vi "Configure Trigger.vi"(8 "error in (no error)":errorcluster, 11 "Thermometer DAQmx Base CFG in":refnum<class "Thermometer DAQmx Base CFG.lvclass">) -> (0 "error out":errorcluster, 3 "Thermometer DAQmx Base CFG out":refnum<class "Thermometer DAQmx Base CFG.lvclass">)   [LabVIEW 2023, in "Thermometer DAQmx Base CFG.lvlib" / "Thermometer DAQmx Base CFG.lvclass"]
uses:
  Thermometer DAQmx Base CFG.lvclass
  Thermometer DAQmx Base CFG.lvclass/Thermometer DAQmx Base CFG.ctl
  1ef251c9-8369-4278-8302-97e96edc9e10.vi
  <vilib>/ErrorRing/Error Ring.xnode
  <vilib>/JDP Science/JSONtext/JSONtext.lvlib
  <vilib>/Utility/error.llb/Error Cluster From Error Code.vi
  Configuration JSON Base/CFG JSON Base.lvclass
  D:/git/HAL/HAL GOOP4/Configuration JSON Base/CFG JSON Base.lvclass
  D:/git/HAL/HAL GOOP4/Interfaces/IConfigure/IConfigure.lvclass
  D:/git/HAL/HAL GOOP4/Thermometer/Thermometer DAQmx Base CFG/Thermometer DAQmx Base CFG.lvclass
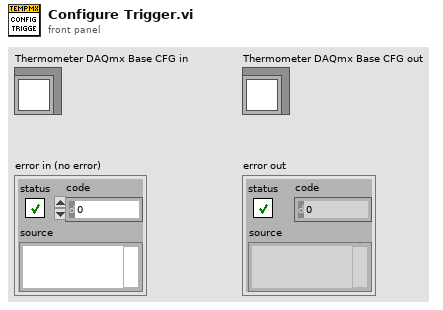
[diagram p1: front panel]
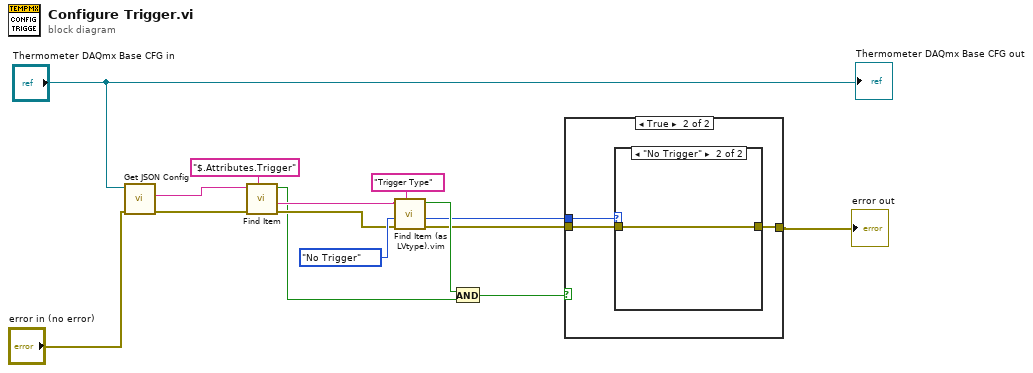
[diagram p0: block diagram]
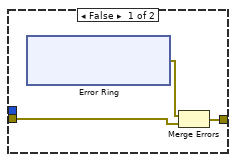
[diagram p2: hidden frame]
diagram:
  n1 = call "Get JSON Config.vi"("error in (no error)"="error in (no error)", "CFG Base in"="Thermometer DAQmx Base CFG in") -> ("error out"=w15:errorcluster, "<JSON>Config>"=w14:string)  [unwired: 7 in, 1 out]
  n2 = call <vilib>:"Find Item.vi"("$Path or Item Name"="$.Attributes.Trigger", "error in (no error)"=w15, "JSON"=w14) -> ("error out"=w8:errorcluster, "<JSON>"=w11:string, "Found"=w7:bool)  [unwired: 5 in, 1 out]
  n3 = call "Find Item (as LVtype).vim"("$Path or Item Name"="Trigger Type", "error in (no error)"=w8, "Data Type and Default Value"=enum16{"No Trigger"}."No Trigger", "JSON"=w11) -> ("error out"=w4:errorcluster, "Data"=w3:enum16{"No Trigger"}, "Found"=w6:bool)  [unwired: 4 in, 1 out]
  n4 = And(x=w6, y=w7) -> (x .and. y?=w5:bool)
  n5 = case shown="True" w5 {
    tunnel: w4 -> [w17 w25]
    tunnel: w3 -> [_ w26]
    tunnel: [w16 w24] -> w2
    frame False {
      n6 = xnode "Error Ring"() -> ("error out"=w18:errorcluster)
      n7 = Merge Errors(w18, w17) -> (w16:errorcluster)
    }
    frame True {
      n8 = case shown="\"No Trigger\"" w26 {
        tunnel: w25 -> [w27 w28]
        tunnel: [w27 w28] -> w24
        frame Default {
        }
        frame "No Trigger" {
        }
      }
    }
  }
  "error out" <- w2
  "Thermometer DAQmx Base CFG out" <- "Thermometer DAQmx Base CFG in"
